vi "request.vi"(0 "Device In":T1, 3 "error in":errorcluster) -> (7 "Device Out":T1, 8 "Comm":T2, 10 "error out":errorcluster)   [LabVIEW 2020]
uses:
  HTTPComm.ctl
  Cluster.ctl
  <vilib>/httpClient/POSTBuffer.vi
  <vilib>/httpClient/LabVIEWHTTPClient.lvlib
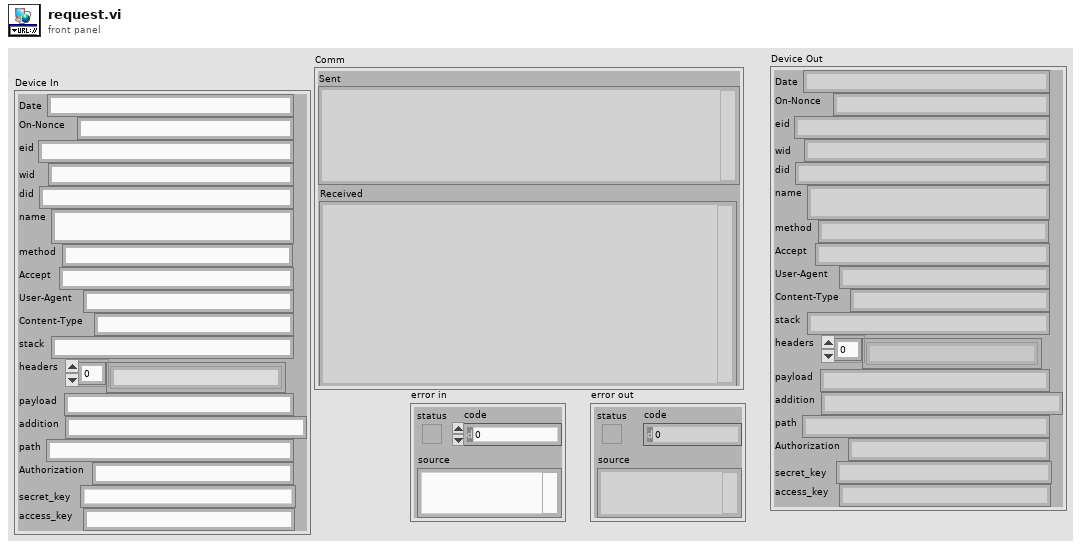
[diagram p1: front panel]
types:
  T1 = typedef "Cluster.ctl" = cluster{"Date":string, "On-Nonce":string, "eid":string, "wid":string, "did":string, "name":string, "method":string, "Accept":string, "User-Agent":string, "Content-Type":string, "stack":string, "headers":string[], "payload":string, "addition":string, "path":string, "Authorization":string, "secret_key":string, "access_key":string}
  T2 = typedef "HTTPComm.ctl" = cluster{"url":string, "sent headers":string, "sent body":string, "headers":string, "body":string, "Sent":string, "Received":string}
  T3 = typedef "LabVIEWHTTPClient.lvlib/ClientHandle.ctl" = refnum<k1>
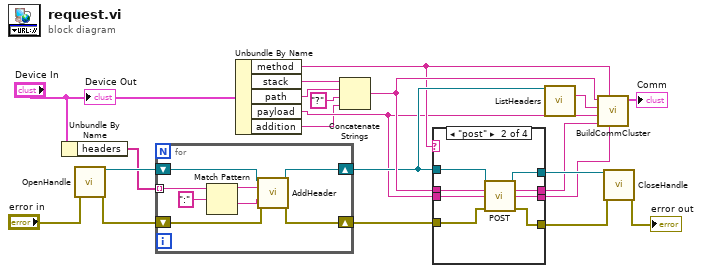
[diagram p0: block diagram]
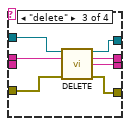
[diagram p3: hidden frame]
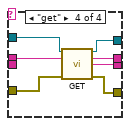
[diagram p4: hidden frame]
diagram:
  n1 = Unbundle By Name("Device In") -> ("headers"=w19:string[])
  n2 = call <vilib>:"OpenHandle.vi"("error in (no error)"="error in") -> ("client handle out"=w20:T3, "error out"=w18:errorcluster)  [unwired: 13 in]
  n3 = for {
    shift-right: [w28] -> w11
    shift-left: w20 -> [w29]
    shift-right: [w26] -> w17
    shift-left: w18 -> [w27]
    tunnel: w19 -> [w22] mode=indexing
    n4 = Match Pattern(string=w22, regular expression=":") -> (before substring=w24:string, after substring=w23:string)  [unwired: 1 in, 2 out]
    n5 = call <vilib>:"AddHeader.vi"("client handle"=w29, "header"=w24, "value"=w23, "error in (no error)"=w27) -> ("client handle out"=w28:T3, "error out"=w26:errorcluster)  [unwired: 10 in]
  }
  n6 = Unbundle By Name("Device In") -> ("method"=w7:string, "stack"=w15:string, "path"=w14:string, "payload"=w6:string, "addition"=w3:string)
  n7 = Concatenate Strings(w15, w14, "?", w3) -> (w12:string)
  n8 = case shown="\"post\"" w7 {
    tunnel: w11 -> [_ w38 w45 w52]
    tunnel: [_ w31 w44 w51] -> w21
    tunnel: [_ w37 w42 w49] -> w8
    tunnel: [_ w36 w43 w50] -> w9
    tunnel: w17 -> [w30 w35 w41 w48]
    tunnel: [w30 w34 w40 w47] -> w2
    tunnel: w12 -> [_ w33 w39 w46]
    tunnel: w6 -> [_ w32 _ _]
    frame Default {
    }
    frame "post" {
      n9 = call-poly <vilib>:"POST.vi"("client handle"=w38, "url"=w33, "buffer"=w32, "error in (no error)"=w35) -> ("client handle out"=w31:T3, "headers"=w36:string, "body"=w37:string, "error out"=w34:errorcluster)  [unwired: 8 in]
    }
    frame "delete" {
      n10 = call <vilib>:"DELETE.vi"("client handle"=w45, "url"=w39, "error in (no error)"=w41) -> ("client handle out"=w44:T3, "headers"=w43:string, "body"=w42:string, "error out"=w40:errorcluster)  [unwired: 9 in]
    }
    frame "get" {
      n11 = call <vilib>:"GET.vi"("client handle"=w52, "url"=w46, "error in (no error)"=w48) -> ("client handle out"=w51:T3, "headers"=w50:string, "body"=w49:string, "error out"=w47:errorcluster)  [unwired: 9 in]
    }
  }
  n12 = call <vilib>:"ListHeaders.vi"("client handle"=w11) -> ("headers"=w10:string)  [unwired: 12 in, 2 out]
  n13 = call "BuildCommCluster.vi"("reply body"=w8, "Type"=w7, "reply headers"=w9, "sent body"=w6, "sent headers"=w10, "url"=w12) -> ("Comm"=→"Comm":T2)  [unwired: 5 in]
  n14 = call <vilib>:"CloseHandle.vi"("client handle"=w21, "error in (no error)"=w2) -> ("error out"=→"error out":errorcluster)  [unwired: 13 in]
  "Device Out" <- "Device In"
